vi "Thermal_Camera_ArrayTempExtract.vi"(8 "error in (no error)":errorcluster, 9 "Mouse pos":cluster{"X":i32, "Y":i32}, 11 "img in":T1) -> (0 "error out":errorcluster, 1 "Mouse pos dup":cluster{"X":i32, "Y":i32}, 2 "temp str":string, 3 "temp":dbl)   [LabVIEW 2020]
uses:
  <vilib>/vision/Image Controls.llb/IMAQ Image.ctl
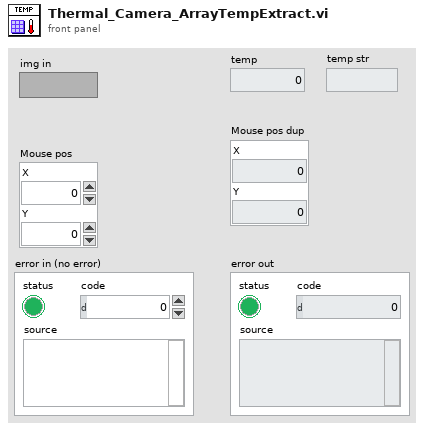
[diagram p1: front panel]
types:
  T1 = typedef "IMAQ Image.ctl" = refnum<image>
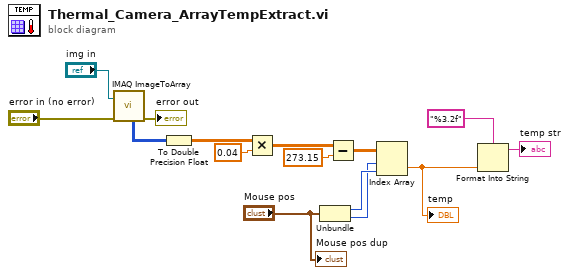
[diagram p0: block diagram]
diagram:
  n1 = call "IMAQ ImageToArray"("error in (no error)"="error in (no error)", "Image"="img in") -> ("Image Pixels (U16)"=w5:u16[][], "error out"=→"error out":errorcluster)  [unwired: 2 in, 3 out]
  n2 = To Double Precision Float(number=w5) -> (double precision float=w8:dbl[][])
  n3 = Multiply(x=w8, y=0.04) -> (x*y=w9:dbl[][])
  n4 = Unbundle("Mouse pos") -> ("X"=w14:i32, "Y"=w13:i32)
  n5 = Subtract(x=w9, y=273.15) -> (x-y=w11:dbl[][])
  n6 = Index Array(array=w11, index (row)=w13, index (col)=w14) -> (element=w1:dbl)
  "temp" <- w1
  n7 = Format Into String(format string="%3.2f", w1) -> (resulting string=→"temp str":string)  [unwired: 2 in, 1 out]
  "Mouse pos dup" <- "Mouse pos"
